vi "Configure DI Module.vi"(0 "VISA resource name":refnum<visa-resource-name>, 1 "Enable Chattering Filter? (0: Not Change)":u16(ring) items=["Not Change", "Off", "On"], 5 "Unit Number (0)":i32 min=0 max=6 step=1, 7 "Module Number (0)":i32 min=0 max=9 step=1, 9 "Operation Mode (0: Normal)":u16(ring) items=["Normal", "Remote"], 11 "error in (no error)":errorcluster) -> (4 "VISA resource name out":refnum<visa-resource-name>, 6 "Unit Number":i32, 8 "Module Number":i32, 15 "error out":errorcluster)   [LabVIEW 2020, in "Yokogawa GX Series.lvlib"]
doc: "Sets operation mode of DI module.\n\nOnly one module can be set \"Remote\" mode. If multiple module are set, the module set at last can be set Remote mode.\n\nCommand: SModeDI"
uses:
  <instrlib>/Yokogawa GX Series/Yokogawa GX Series.lvlib
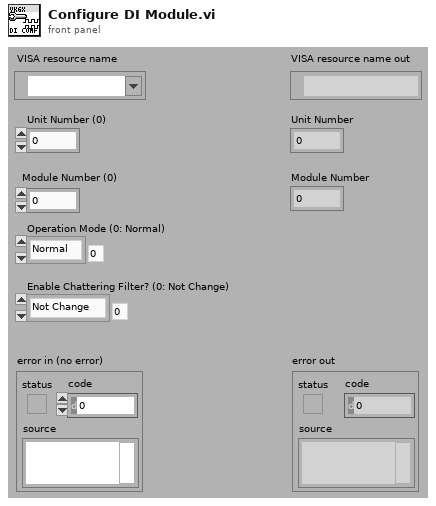
[diagram p1: front panel]
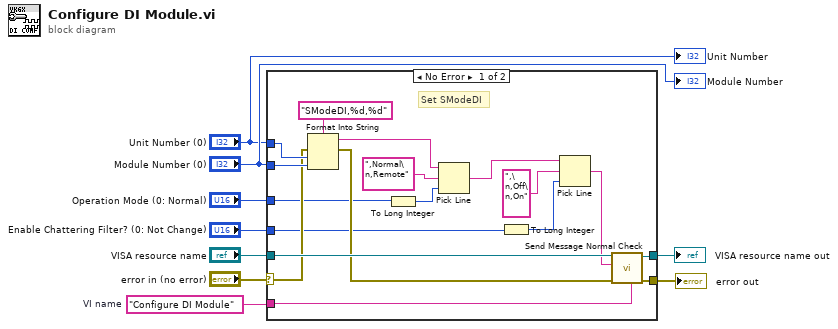
[diagram p0: block diagram]
diagram:
  w2 = "Configure DI Module"  # VI name
  n1 = case shown="No Error" "error in (no error)" {
    selector: "error in (no error)" -> [w18 w29]
    tunnel: "VISA resource name" -> [w26 w28]
    tunnel: [w24 w28] -> w8
    tunnel: [w23 w29] -> w7
    tunnel: "Operation Mode (0: Normal)" -> [w10 _]
    tunnel: "Unit Number (0)" -> [w20 _]
    tunnel: "Module Number (0)" -> [w19 _]
    tunnel: w2 -> [w17 _]
    tunnel: "Enable Chattering Filter? (0: Not Change)" -> [w13 _]
    frame No Error {
      # "Set SModeDI"
      n2 = Format Into String(format string="SModeDI,%d,%d", error in=w18, w20, w19) -> (resulting string=w22:string, error out=w25:errorcluster)  [unwired: 1 in]
      n3 = To Long Integer(number=w10) -> (32bit integer=w11:i32)
      n4 = Pick Line(string ("")=w22, multi-line string=",Normal\n,Remote", line index=w11) -> (output string=w16:string)
      n5 = To Long Integer(number=w13) -> (32bit integer=w12:i32)
      n6 = Pick Line(string ("")=w16, multi-line string=",\n,Off\n,On", line index=w12) -> (output string=w14:string)
      n7 = call <instrlib>:"Send Message Normal Check.vi"("Source (\"\")"=w17, "error in (no error)"=w25, "Send Message (\"\")"=w14, "VISA resource name"=w26) -> ("error out"=w23:errorcluster, "VISA resource name out"=w24:refnum<visa-resource-name>)  [unwired: 2 in, 4 out]
    }
    frame Error {
    }
  }
  "error out" <- w7
  "VISA resource name out" <- w8
  "Unit Number" <- "Unit Number (0)"
  "Module Number" <- "Module Number (0)"
